vi "EX7-3_Tone.vi"() -> ()   [LabVIEW 2012, in "LabVIEW Interface for Arduino.lvlib"]
doc: "An example that uses the arduino's digital output pins to generate a tone that can be played on a speaker or piezo buzzer."
uses:
  <vilib>/LabVIEW Interface for Arduino/LabVIEW Interface for Arduino.lvlib
panel:
  in  "Stop":bool
  in  "Duration ms":u32=1
  in  "Frequency":u16=500 step=100
  in  "Tone DO Pin":u8=8
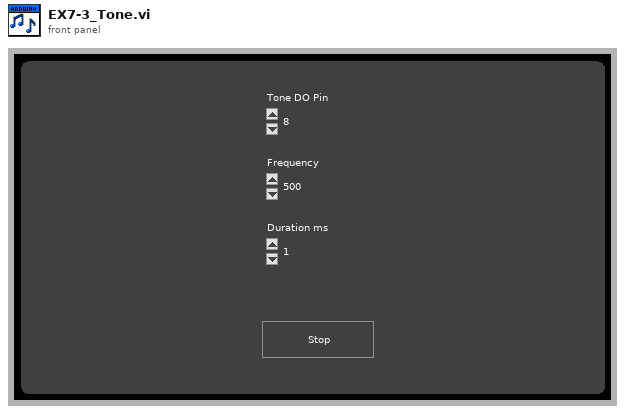
[diagram p1: front panel]
types:
  T1 = typedef "LabVIEW Interface for Arduino.lvlib/Arduino Resource.ctl" = cluster{"VISA resource":refnum<visa-resource-name>, "Board Type":T2, "Connection Type":enum8{"USB / Serial"}, "Bytes Per Packet (15)":u8}
  T2 = typedef "LabVIEW Interface for Arduino.lvlib/Board Type.ctl" = enum16{"Uno", "Dimuelanove w/Atmega 328", "Mega 2560"}
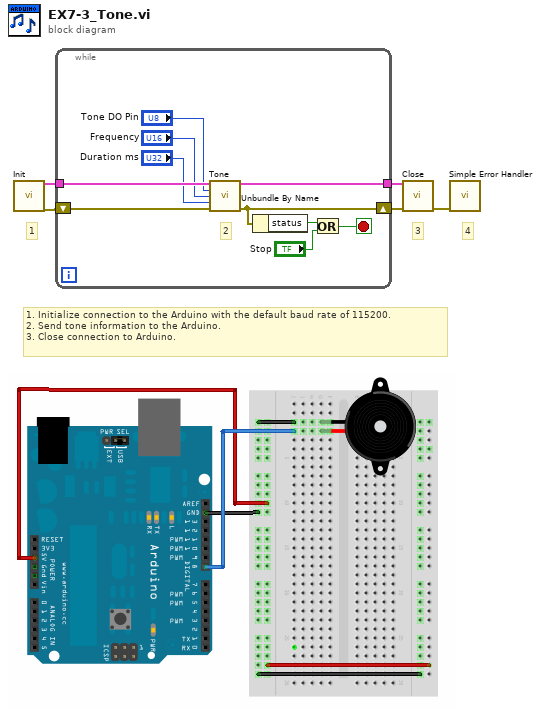
[diagram p0: block diagram]
diagram:
  # "1. Initialize connection to the Arduino with the default baud rate of 115200.\n2. Send tone information to the Arduino.\n3. Close connection to Arduino."
  # "4"
  # "3"
  # "1"
  n1 = call <vilib>:"Init.vi"() -> ("Arduino Resource"=w5:T1, "error out"=w4:errorcluster)  [unwired: 18 in]
  n2 = while {
    tunnel: w5 -> [w13]
    shift-right: [w10] -> w3
    shift-left: w4 -> [w12]
    tunnel: [w11] -> w2
    stop <- w15 stop-if-true
    # "2"
    n3 = call <vilib>:"Tone.vi"("Arduino Resource"=w13, "Tone DO Pin"="Tone DO Pin", "Frequency (0 Hz)"="Frequency", "Duration (1 ms)"="Duration ms", "error in"=w12) -> ("Arduino Resource"=w11:T1, "error out"=w10:errorcluster)  [unwired: 9 in]
    n4 = Unbundle By Name(w10) -> ("status"=w14:bool)
    n5 = Or(x=w14, y="Stop") -> (x .or. y?=w15:bool)
  }
  n6 = call <vilib>:"Close.vi"("Arduino Resource"=w2, "error in"=w3) -> ("error out"=w1:errorcluster)  [unwired: 13 in]
  n7 = call <vilib>:"Simple Error Handler.vi"("error in (no error)"=w1) -> ()  [unwired: 4 in, 5 out]
